vi "task_booleanUserEvent.vi"(8 "error in (no error)":errorcluster, 10 "ITaskChannel":refnum<class "ITaskChannel.lvclass">, 11 "ITask in":refnum<class "ITask.lvclass">) -> (0 "error out":errorcluster, 3 "ITask out":refnum<class "ITask.lvclass">)   [LabVIEW 2023]
uses:
  TLC_Daemon.lvlib
  ITask/ITask.lvclass
  ITaskChannel/ITaskChannel.lvclass
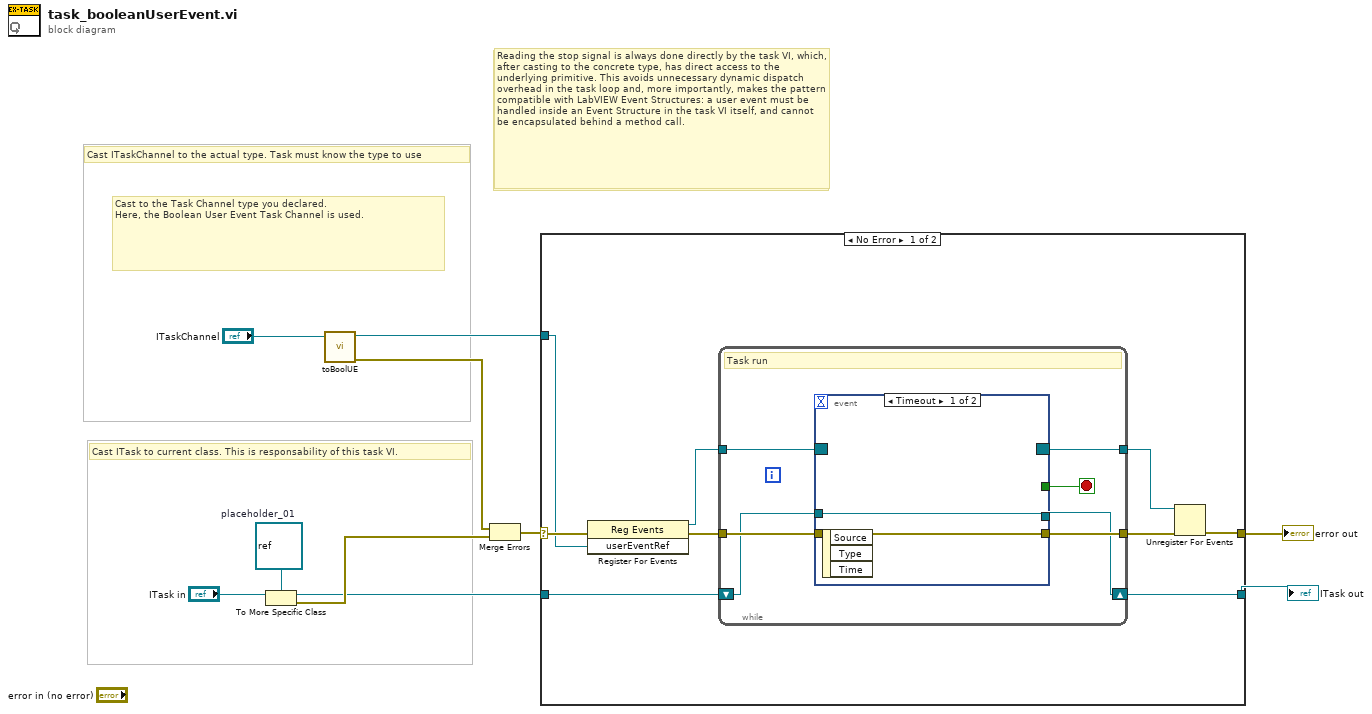
[diagram p0: block diagram]
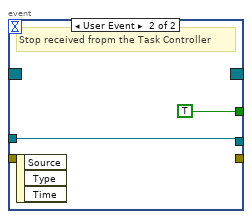
[diagram p2: hidden frame]
diagram:
  w8 = refnum<class> refnum  # placeholder_01
  # "Cast to the Task Channel type you declared.\nHere, the Boolean User Event Task Channel is used."
  # "The stop signal is always handled directly by the task VI, which, after casting to the concrete type, has direct access to the underlying primitive. This avoids unnecessary dynamic dispatch overhead in the task loop and, more importantly, makes the pattern compatible with LabVIEW Event Structures: a user event must be handled inside an Event Structure in the task VI itself, and cannot be encapsulated behind a method call."
  # "Reading the stop signal is always done directly by the task VI, which, after casting to the concrete type, has direct access to the underlying primitive. This avoids unnecessary dynamic dispatch overhead in the task loop and, more importantly, makes the pattern compatible with LabVIEW Event Structures: a user event must be handled inside an Event Structure in the task VI itself, and cannot be encapsulated behind a method call."
  # "Cast ITask to current class. This is responsability of this task VI."
  # "Cast ITaskChannel to the actual type. Task must know the type to use"
  n1 = To More Specific Class(target class=w8, reference="ITask in") -> (specific class reference=w5:refnum<class>, error out=w9:errorcluster)  [unwired: 1 in]
  n2 = call "toBoolUE.vi"("ITaskChannel"="ITaskChannel") -> ("error out"=w1:errorcluster, "userEventRef"=w2:refnum<user-event>)  [unwired: 9 in]
  n3 = Merge Errors(w1, w9) -> (w7:errorcluster)
  n4 = case shown="No Error" w7 {
    selector: w7 -> [w19 w32]
    tunnel: w2 -> [w17 _]
    tunnel: [w14 w32] -> w6
    tunnel: w5 -> [w12 w31]
    tunnel: [w11 w31] -> w4
    frame No Error {
      n5 = register-events(error in=w19, w17) -> (reference out=w16:refnum<event-registration>, error out=w18:errorcluster)  [unwired: 1 in]
      n6 = while {
        tunnel: w18 -> [w26]
        tunnel: [w25] -> w13
        tunnel: w16 -> [w24]
        tunnel: [w22] -> w15
        shift-right: [w20] -> w11
        shift-left: w12 -> [w21]
        stop <- w23 stop-if-true
        # "Task run"
        n7 = event shown="[0] Timeout" {
          selector: w24 -> [_ _]
          dyn-events: [_ _] -> w22
          timeout: _ -> [_ _]
          tunnel: w26 -> [w28 _]
          tunnel: [w28 _] -> w25
          tunnel: [_ TRUE] -> w23
          tunnel: w21 -> [w27 w29]
          tunnel: [w27 w29] -> w20
          event Timeout {
            n8 = event-data() -> ()  [unwired: 1 in, 3 out]
          }
          event User Event {
            # "Stop received fropm the Task Controller"
            n9 = event-data() -> ()  [unwired: 1 in, 3 out]
          }
        }
      }
      n10 = Unregister For Events(event registration refnum=w15, error in=w13) -> (error out=w14:errorcluster)
    }
    frame Error {
    }
  }
  "error out" <- w6
  "ITask out" <- w4
